vi "MotionProfile.vi"(8 "Right":T1={"DeviceStatus"={"status"=FALSE, "code"=0, "source"=""}, "Type"=enum."PWM", "PWM"={"PWM Channel"=enum."Invalid", "DeadBand"={"Name"="", "maxPositivePwm"=0, "minPositivePwm"=0, "centerPwm"=0, "maxNegativePwm"=0, "minNegativePwm"=0, "angularRange"=0}}, "CAN"={"Device Number"=0, "SetOutput VI Ref"=variant(refnum<vi> refnum), "GetOutput VI Ref"=variant(refnum<vi> refnum), "Enable VI Ref"=variant(refnum<vi> refnum), "Disable VI Ref"=variant(refnum<vi> refnum), "Data"=variant}, "Invert"=FALSE, "DIO PWM"={"PWM \"Enable\" Channel"=enum."Invalid", "DIOChannel"=enum."Invalid", "PWM Rate"=0.0}}, 10 "file name":string, 11 "Left":T1={"DeviceStatus"={"status"=FALSE, "code"=0, "source"=""}, "Type"=enum."PWM", "PWM"={"PWM Channel"=enum."Invalid", "DeadBand"={"Name"="", "maxPositivePwm"=0, "minPositivePwm"=0, "centerPwm"=0, "maxNegativePwm"=0, "minNegativePwm"=0, "angularRange"=0}}, "CAN"={"Device Number"=0, "SetOutput VI Ref"=variant(refnum<vi> refnum), "GetOutput VI Ref"=variant(refnum<vi> refnum), "Enable VI Ref"=variant(refnum<vi> refnum), "Disable VI Ref"=variant(refnum<vi> refnum), "Data"=variant}, "Invert"=FALSE, "DIO PWM"={"PWM \"Enable\" Channel"=enum."Invalid", "DIOChannel"=enum."Invalid", "PWM Rate"=0.0}}) -> ()   [LabVIEW 2019]
uses:
  <vilib>/Rock Robotics/WPI/MotorControl/WPI_MotorControlDeviceRef.ctl
  <vilib>/Rock Robotics/WPI/MotorControl/WPI_MotorControlType.ctl
  <vilib>/Rock Robotics/SystemInterfaces/DIO/FPGA_DIOPWMChannel.ctl
  <vilib>/Rock Robotics/WPI/PWM/WPI_PWMDeadband.ctl
  <vilib>/Rock Robotics/SystemInterfaces/DIO/FPGA_DIOChannel.ctl
  Motion_Profiler_Class/MotionProfiles.lvclass
  <vilib>/Rock Robotics/WPI/ThirdParty/Phoenix-LabVIEW/CANCoder/Set/CTRE_Phoenix_CANcoder_SetPosition.vi
panel:
  out "start2":bool
  out "start":bool
  out "Left Motor":T6(graph)
  out "Left Throttle":dbl(graph)
  out "Right Motor":T7(graph)
  out "Right Throttle":dbl(graph)
  out "Right Bottom Buf Count":i32
  out "Left Bottom Buf Count":i32
  out "Right Under Run":bool
  out "Left Under Run":bool
  out "Set_Vel_(u/100ms)":i32
  out "Set_Pos_(u)":i32
  out "Act_Vel_(u/100ms)":i32
  out "Act_Pos(u)":i32
  out "MP Is Executing":bool
  out "Motion Profile Status":T8
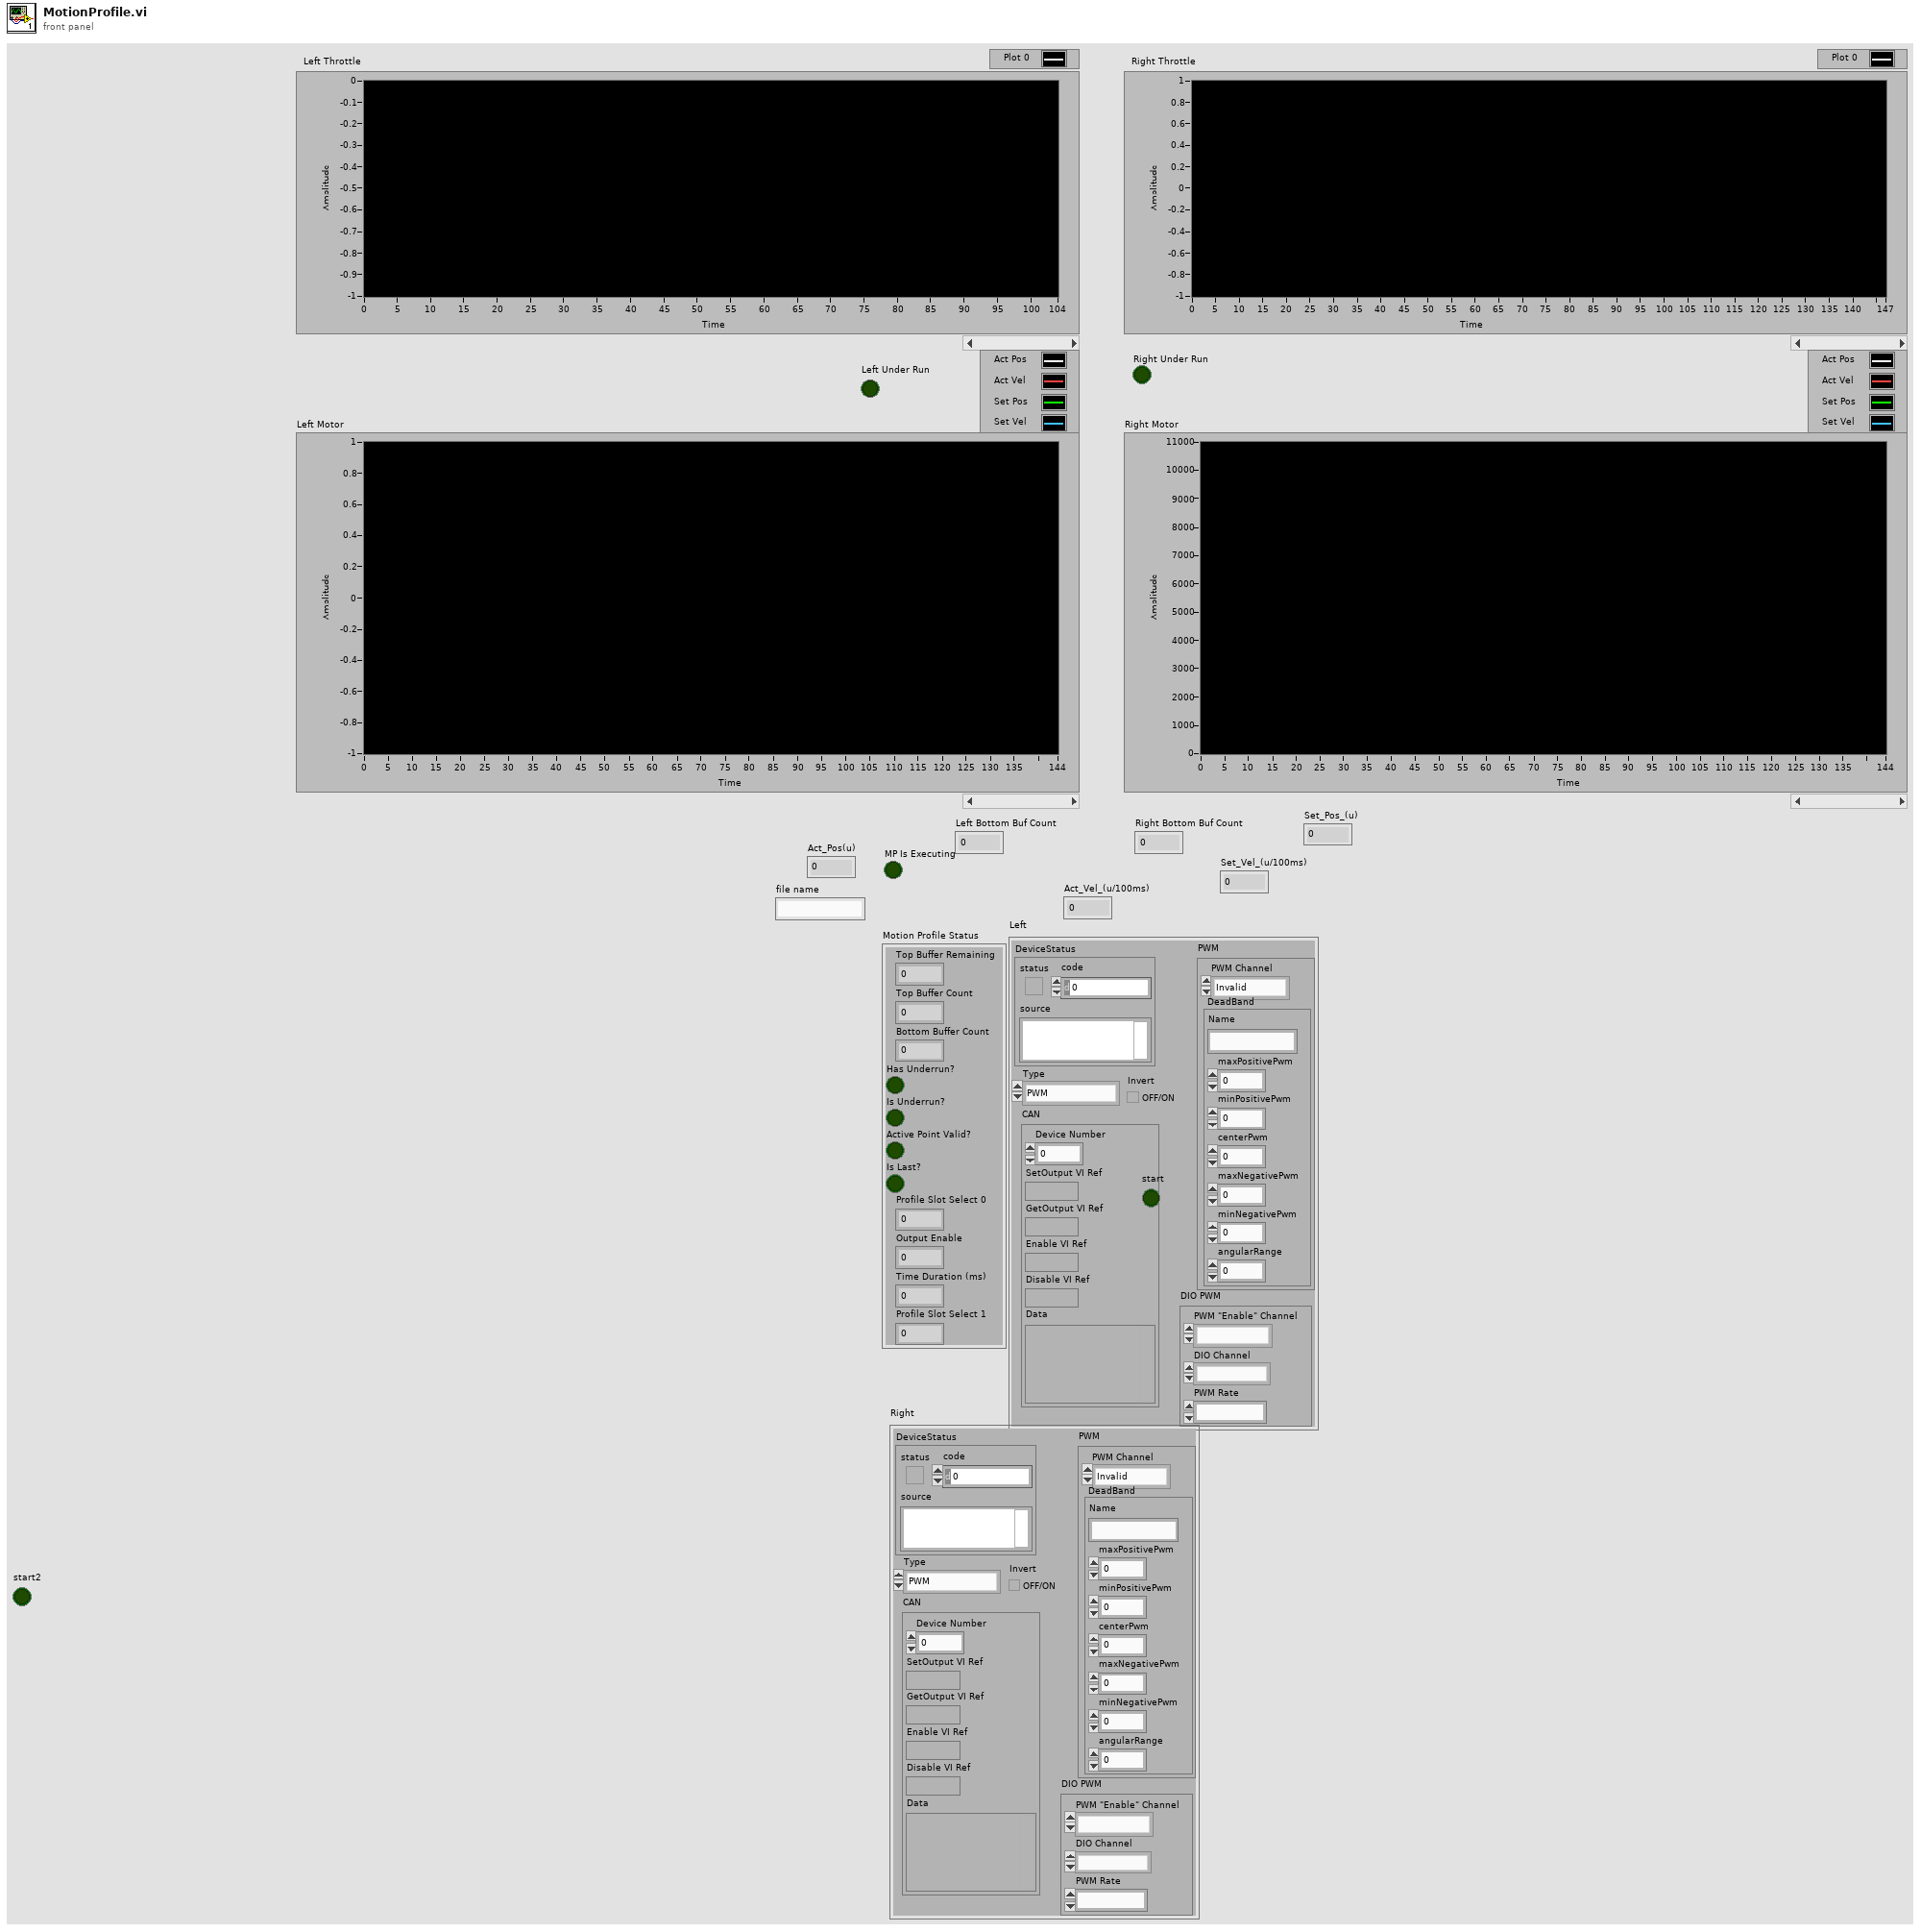
[diagram p1: front panel]
types:
  T1 = typedef "WPI_MotorControlDeviceRef.ctl" = cluster{"DeviceStatus":errorcluster, "Type":T2, "PWM":cluster{"PWM Channel":T3, "DeadBand":T4}, "CAN":cluster{"Device Number":u8, "SetOutput VI Ref":variant, "GetOutput VI Ref":variant, "Enable VI Ref":variant, "Disable VI Ref":variant, "Data":variant}, "Invert":bool, "DIO PWM":cluster{"PWM \"Enable\" Channel":T3, "DIOChannel":T5, "PWM Rate":dbl}}
  T2 = typedef "WPI_MotorControlType.ctl" = enum16{"PWM", "CAN", "DIO PWM"}
  T3 = typedef "FPGA_DIOPWMChannel.ctl" = enum8{"PWM 0", "PWM 1", "PWM 2", "PWM 3", "PWM 4", "PWM 5", "PWM 6", "PWM 7", "PWM 8", "PWM 9", "PWM MXP 0", "PWM MXP 1", "PWM MXP 2", "PWM MXP 3", "PWM MXP 4", "PWM MXP 5", "PWM MXP 6", "PWM MXP 7", "PWM MXP 8", "PWM MXP 9", "Invalid"}
  T4 = typedef "WPI_PWMDeadband.ctl" = cluster{"Name":string, "maxPositivePwm":i32, "minPositivePwm":i32, "centerPwm":i32, "maxNegativePwm":i32, "minNegativePwm":i32, "angularRange":u16}
  T5 = typedef "FPGA_DIOChannel.ctl" = enum8{"DIO 0", "DIO 1", "DIO 2", "DIO 3", "DIO 4", "DIO 5", "DIO 6", "DIO 7", "DIO 8", "DIO 9", "DIO MXP 0", "DIO MXP 1", "DIO MXP 2", "DIO MXP 3", "DIO MXP 4", "DIO MXP 5", "DIO MXP 6", "DIO MXP 7", "DIO MXP 8", "DIO MXP 9", "DIO MXP 10", "DIO MXP 11", "DIO MXP 12", "DIO MXP 13", "DIO MXP 14", "DIO MXP 15", "SPI Port CS1", "SPI Port CS2", "SPI Port CS3", "SPI Port MISO", "SPI Port MOSI", "Invalid"}
  T6 = cluster{"Set_Pos_(u)":i32, "Set_Pos_(u)":i32, "Act_Vel_(u/100ms)":i32, "Set_Vel_(u/100ms)":i32}
  T7 = cluster{"Set_Vel_(u/100ms)":i32, "Act_Vel_(u/100ms)":i32, "Set_Pos_(u)":i32, "Act_Pos(u)":i32}
  T8 = cluster{"Top Buffer Remaining":i32, "Top Buffer Count":i32, "Bottom Buffer Count":i32, "Has Underrun?":bool, "Is Underrun?":bool, "Active Point Valid?":bool, "Is Last?":bool, "Profile Slot Select 0":i32, "Output Enable":i32, "Time Duration (ms)":i32, "Profile Slot Select 1":i32}
  T9 = typedef "CTRE_Phoenix_CANcoder_DeviceRef.ctl" = cluster{"DeviceStatus":errorcluster, "Device Number":u8, "Handle":u64, "UsageFrame":u32, "Library Path":path}
  T10 = typedef "MotionProfiles.lvclass/MotionProfile_MP_Class_Status.ctl" = cluster{"Motion Profile Status":cluster{"Top Buffer Remaining":i32, "Top Buffer Count":i32, "Bottom Buffer Count":i32, "Has Underrun?":bool, "Is Underrun?":bool, "Active Point Valid?":bool, "Is Last?":bool, "Profile Slot Select 0":i32, "Output Enable":i32, "Time Duration (ms)":i32, "Profile Slot Select 1":i32}, "TalonState":T11, "MP Is Done":bool, "MP Is Executing":bool, "Set_Vel_(u/100ms)":i32, "Set_Pos_(u)":i32, "Act_Vel_(u/100ms)":i32, "Act_Pos(u)":i32, "Throtle":dbl}
  T11 = typedef "MotionProfiles.lvclass/MotionProfile_TalonSetValueEnum.ctl" = enum16{"Disable", "Enable", "Hold"}
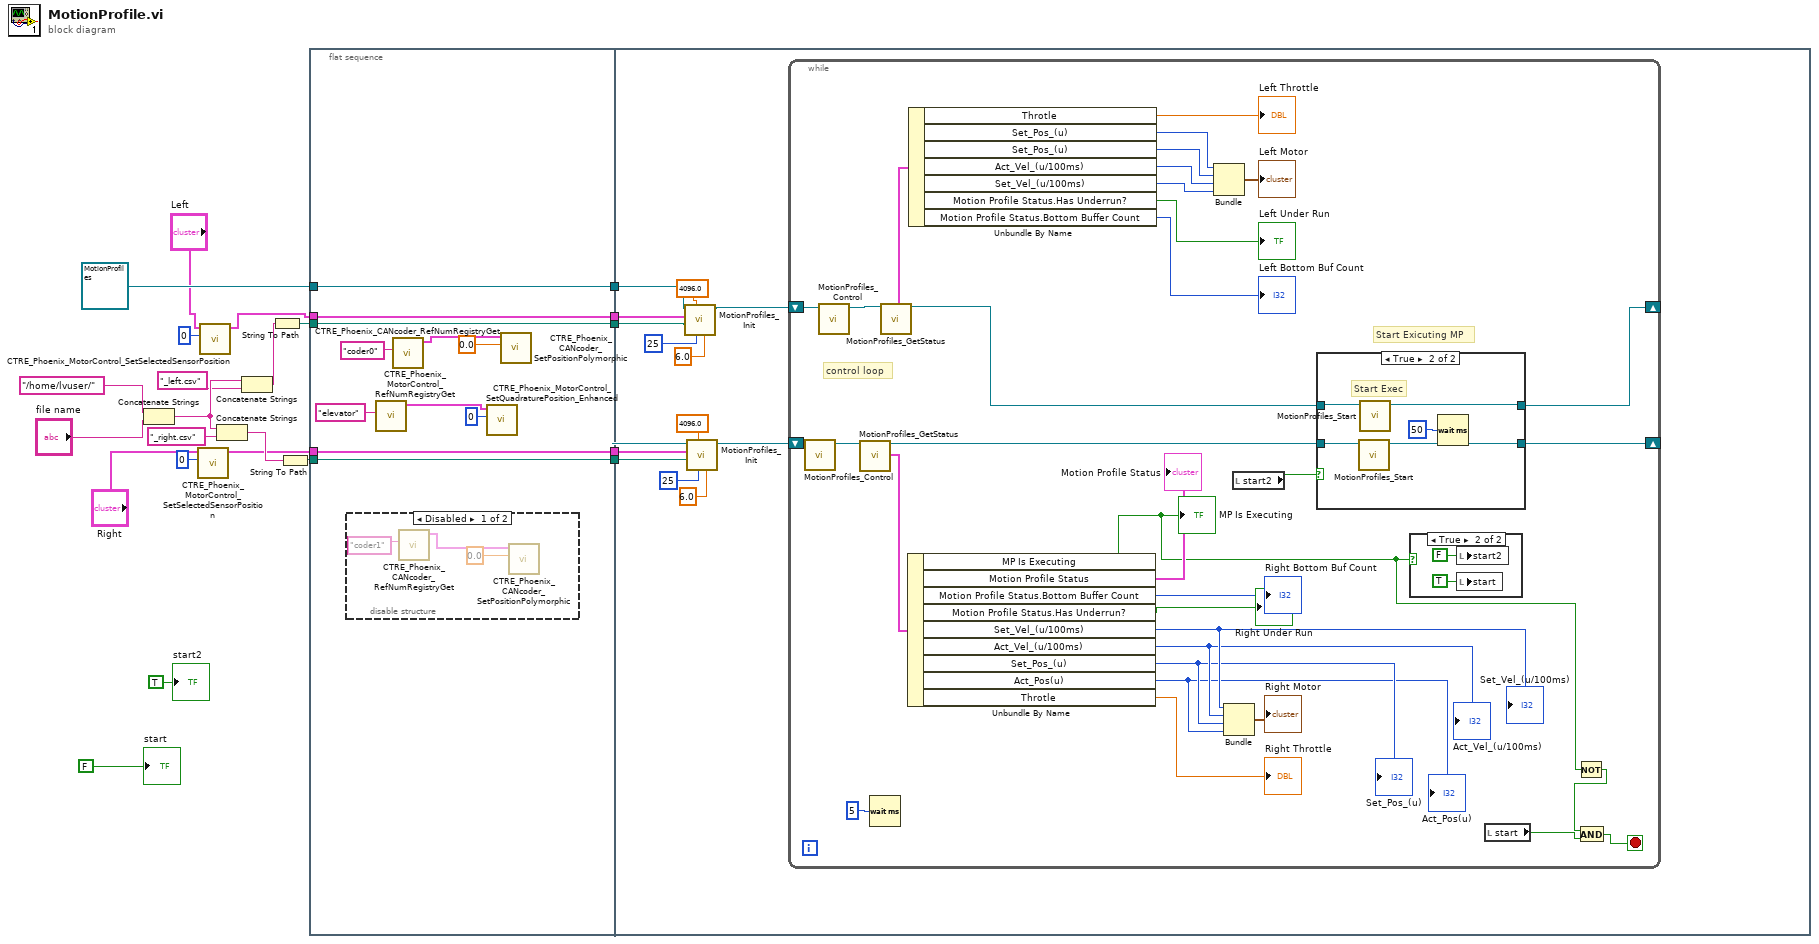
[diagram p0: block diagram]
diagram:
  n1 = Concatenate Strings("/home/lvuser/", "file name") -> (w17:string)
  n2 = call <vilib>:"CTRE_Phoenix_MotorControl_SetSelectedSensorPosition.vi"("New Sensor Position"=0, "PhoenixMotorControlDevRef"="Right") -> ("PhoenixMotorControlDevRef"=w10:T1)  [unwired: 8 in, 1 out]
  n3 = call <vilib>:"CTRE_Phoenix_MotorControl_SetSelectedSensorPosition.vi"("New Sensor Position"=0, "PhoenixMotorControlDevRef"="Left") -> ("PhoenixMotorControlDevRef"=w6:T1)  [unwired: 8 in, 1 out]
  n4 = Concatenate Strings(w17, "_right.csv") -> (w19:string)
  n5 = Concatenate Strings(w17, "_left.csv") -> (w15:string)
  n6 = String To Path(string=w15) -> (path=w14:path)
  n7 = String To Path(string=w19) -> (path=w18:path)
  n8 = flat-sequence {
    tunnel: w6 -> [w30]
    tunnel: w10 -> [w31]
    tunnel: w14 -> [w32]
    tunnel: w18 -> [w33]
    tunnel: refnum<class "MotionProfiles.lvclass"> refnum ("MotionProfiles.lvclass") -> [w34]
    tunnel: [w34] -> w5
    tunnel: [w33] -> w4
    tunnel: [w32] -> w3
    tunnel: [w31] -> w2
    tunnel: [w30] -> w1
    tunnel: w5 -> [w48]
    tunnel: w4 -> [w41]
    tunnel: w3 -> [w40]
    tunnel: w2 -> [w39]
    tunnel: w1 -> [w38]
    frame #0 {
      n9 = disable-structure shown="Disabled" {
        frame Disabled {
          n10 = call <vilib>:"CTRE_Phoenix_CANcoder_RefNumRegistryGet.vi"("refnum name"="coder1") -> ("CTRE_CANcoder_DeviceRef"=w36:T9)  [unwired: 9 in, 1 out]
          n11 = call-poly <vilib>:"CTRE_Phoenix_CANcoder_SetPositionPolymorphic.vi"("Position"=0.0, "CTRE_CANcoder_DeviceRef"=w36) -> ()  [unwired: 8 in, 2 out]
        }
        frame Enabled {
        }
      }
      n12 = call <vilib>:"CTRE_Phoenix_MotorControl_RefNumRegistryGet.vi"("refnum name"="elevator") -> ("PhoenixMotorControlDevRef"=w25:T1)  [unwired: 9 in, 1 out]
      n13 = call <vilib>:"CTRE_Phoenix_CANcoder_RefNumRegistryGet.vi"("refnum name"="coder0") -> ("CTRE_CANcoder_DeviceRef"=w28:T9)  [unwired: 9 in, 1 out]
      n14 = call <vilib>:"CTRE_Phoenix_MotorControl_SetQuadraturePosition_Enhanced.vi"("New Position"=0, "PhoenixMotorControlDevRef"=w25) -> ()  [unwired: 8 in, 2 out]
      n15 = call-poly <vilib>:"CTRE_Phoenix_CANcoder_SetPositionPolymorphic.vi"("Position"=0.0, "CTRE_CANcoder_DeviceRef"=w28) -> ()  [unwired: 8 in, 2 out]
    }
    frame #1 {
      n16 = call "MotionProfiles_Init.vi"("Wheel_Diameter (in)"=6.0 ("Wheel Diameter"), "MP_Frame_Rate_(ms)"=25, "Encoder_CPR_4x"=4096.0, "CSV File Path"=w40, "PhoenixMotorControlDevRef"=w38, "MotionProfiles in"=w48) -> ("MotionProfiles out"=w50:refnum<class "MotionProfiles.lvclass">)  [unwired: 3 in, 2 out]
      n17 = call "MotionProfiles_Init.vi"("Wheel_Diameter (in)"=6.0, "MP_Frame_Rate_(ms)"=25, "Encoder_CPR_4x"=4096.0, "CSV File Path"=w41, "PhoenixMotorControlDevRef"=w39, "MotionProfiles in"=w48) -> ("MotionProfiles out"=w49:refnum<class "MotionProfiles.lvclass">)  [unwired: 3 in, 2 out]
      n18 = while {
        shift-right: [w79] -> _
        shift-left: w50 -> [w82]
        shift-right: [w80] -> _
        shift-left: w49 -> [w81]
        stop <- w54 stop-if-true
        # "control loop"
        # "Start Exicuting MP"
        n19 = call "MotionProfiles_Control.vi"("MotionProfiles in"=w81) -> ("MotionProfiles out"=w76:refnum<class "MotionProfiles.lvclass">)  [unwired: 9 in, 1 out]
        n20 = call "MotionProfiles_Control.vi"("MotionProfiles in"=w82) -> ("MotionProfiles out"=w77:refnum<class "MotionProfiles.lvclass">)  [unwired: 9 in, 1 out]
        n21 = call "MotionProfiles_GetStatus.vi"("MotionProfiles in"=w76) -> ("MotionProfiles out"=w59:refnum<class "MotionProfiles.lvclass">, "MP_Class_Status"=w75:T10)  [unwired: 12 in, 1 out]
        n22 = Wait (ms)(milliseconds to wait=u32 5) -> ()  [unwired: 1 out]
        n23 = call "MotionProfiles_GetStatus.vi"("MotionProfiles in"=w77) -> ("MotionProfiles out"=w78:refnum<class "MotionProfiles.lvclass">, "MP_Class_Status"=w68:T10)  [unwired: 12 in, 1 out]
        n24 = Unbundle By Name(w75) -> ("MP Is Executing"=w51:bool, "Motion Profile Status"=→"Motion Profile Status":T8, "Motion Profile Status.Bottom Buffer Count"=→"Right Bottom Buf Count":i32, "Motion Profile Status.Has Underrun?"=→"Right Under Run":bool, "Set_Vel_(u/100ms)"=w72:i32, "Act_Vel_(u/100ms)"=w71:i32, "Set_Pos_(u)"=w70:i32, "Act_Pos(u)"=w58:i32, "Throtle"=→"Right Throttle":dbl)
        "Set_Vel_(u/100ms)" <- w72
        "Set_Pos_(u)" <- w70
        "Act_Vel_(u/100ms)" <- w71
        "Act_Pos(u)" <- w58
        "MP Is Executing" <- w51
        n25 = Unbundle By Name(w68) -> ("Throtle"=→"Left Throttle":dbl, "Set_Pos_(u)"=w61:i32, "Set_Pos_(u)"=w62:i32, "Act_Vel_(u/100ms)"=w63:i32, "Set_Vel_(u/100ms)"=w64:i32, "Motion Profile Status.Has Underrun?"=→"Left Under Run":bool, "Motion Profile Status.Bottom Buffer Count"=→"Left Bottom Buf Count":i32)
        n26 = Bundle("Set_Pos_(u)"=w61, "Set_Pos_(u)"=w62, "Act_Vel_(u/100ms)"=w63, "Set_Vel_(u/100ms)"=w64) -> (→"Left Motor":T6)  [unwired: 1 in]
        n27 = Bundle("Set_Vel_(u/100ms)"=w72, "Act_Vel_(u/100ms)"=w71, "Set_Pos_(u)"=w70, "Act_Pos(u)"=w58) -> (→"Right Motor":T7)  [unwired: 1 in]
        n28 = local read "start2"() -> (w56:bool)
        n29 = case shown="True" w56 {
          tunnel: w78 -> [w87 w92]
          tunnel: w59 -> [w86 w90]
          tunnel: [w86 w89] -> w80
          tunnel: [w87 w91] -> w79
          frame False {
          }
          frame True {
            # "Start Exec"
            n30 = call "MotionProfiles_Start.vi"("MotionProfiles in"=w90) -> ("MotionProfiles out"=w89:refnum<class "MotionProfiles.lvclass">)  [unwired: 9 in, 1 out]
            n31 = call "MotionProfiles_Start.vi"("MotionProfiles in"=w92) -> ("MotionProfiles out"=w91:refnum<class "MotionProfiles.lvclass">)  [unwired: 9 in, 1 out]
            n32 = Wait (ms)(milliseconds to wait=u32 50) -> ()  [unwired: 1 out]
          }
        }
        n33 = case shown="True" w51 {
          frame False {
          }
          frame True {
            n34 = local write "start2"(FALSE ("start2")) -> ()
            n35 = local write "start"(TRUE ("start")) -> ()
          }
        }
        n36 = local read "start"() -> (w53:bool)
        n37 = Not(x=w51) -> (.not. x?=w52:bool)
        n38 = And(x=w52, y=w53) -> (x .and. y?=w54:bool)
      }
    }
  }
  "start" <- FALSE ("start")
  "start2" <- TRUE ("start2")
